vi "Add Object.vi"(8 "error in (no error)":errorcluster, 10 "Object":refnum<class "Service.lvclass">, 11 "Arguments in":refnum<class "Arguments.lvclass">) -> (0 "error out":errorcluster, 3 "Arguments out":refnum<class "Arguments.lvclass">)   [LabVIEW 2020]
uses:
  Arguments.lvclass/Arguments.ctl
  <vilib>/Utility/miscctls.llb/LVMapReplaceAction.ctl
  <vilib>/ErrorRing/Error Ring.xnode
  <vilib>/Utility/error.llb/Error Cluster From Error Code.vi
  d39a5ae9-4cf2-42c9-b8ff-cb9f4578f042.vi
  Arguments.lvclass
  Service/Service.lvclass
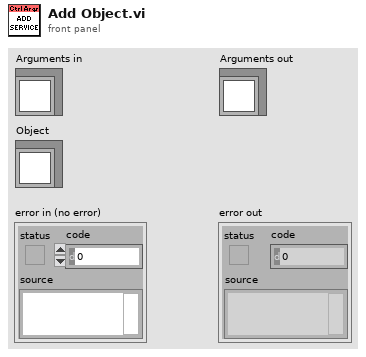
[diagram p1: front panel]
types:
  T1 = typedef "LVMapReplaceAction.ctl" = enum32{"Modify Entry only if found", "Add or Modify Entry", "Delete Entry"}
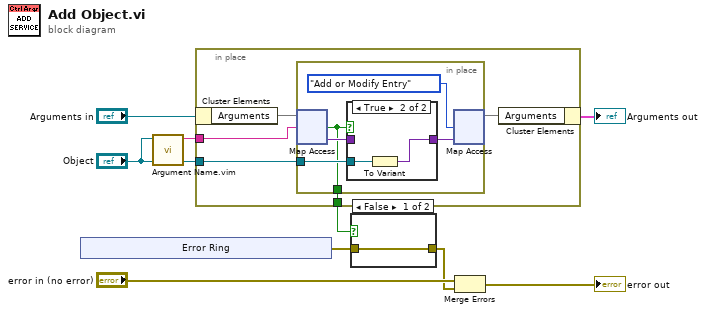
[diagram p0: block diagram]
diagram:
  n1 = xnode "Error Ring"() -> ("error out"=w6:errorcluster)
  n2 = call "Argument Name.vim"("Object / Name"="Object") -> ("Service Key"=w2:string)  [unwired: 8 in, 2 out]
  n3 = in-place {
    in-place-border: w2 -> [w13]
    in-place-border: "Object" -> [w12]
    in-place-border: [w10] -> w7
    n4 = in-place-cluster #1("Arguments in") -> ("Arguments"=w14)
    n5 = in-place {
      in-place-border: w12 -> [w17]
      in-place-border: [w15] -> w10
      n6 = in-place-map #2(w14, w13) -> (w18:variant, w15:bool)  [unwired: 1 in]
      n7 = case shown="True" w15 {
        tunnel: w18 -> [w20 _]
        tunnel: w17 -> [_ w22]
        tunnel: [w20 w21] -> w16
        frame False {
        }
        frame True {
          n8 = To Variant(anything=w22) -> (Variant=w21:variant)
        }
      }
      n9 = in-place-map #2(w16, LVMapReplaceAction."Add or Modify Entry" ("action")) -> (w11:map{string, variant})  [unwired: 2 out]
    }
    n10 = in-place-cluster #1("Arguments"=w11) -> (→"Arguments out":cluster{})
  }
  n11 = case shown="False" w7 {
    tunnel: w6 -> [w23 _]
    tunnel: [w23 _] -> w4
    frame False {
    }
    frame True {
    }
  }
  n12 = Merge Errors("error in (no error)", w4) -> (→"error out":errorcluster)
